vi "delLastComma.vi"(11 "字符串":string) -> (3 "result string":string)   [LabVIEW 2011]
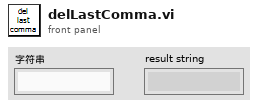
[diagram p1: front panel]
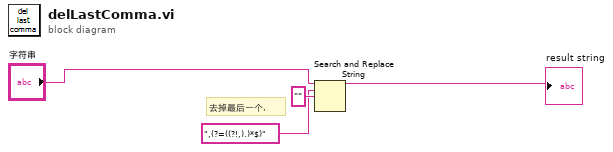
[diagram p0: block diagram]
diagram:
  # "去掉最后一个,"
  n1 = Search and Replace String(input string="字符串", search string=",(?=((?!,).)*$)" ("搜索字符串"), replace string="" ("替换字符串(\"\")")) -> (result string=→"result string":string)  [unwired: 5 in, 3 out]
